vi "solar Destroy (Targets).vi"(8 "error in (no error)":errorcluster, 11 "TargetVIs":refnum<vi>[](array[refnum])) -> (0 "error out":errorcluster)   [LabVIEW 2018]
doc: "This collects all child target VIs before closing the application. This ensures all references generated by the targets are properly destroyed."
panel:
  out "VI":string
  out "VIs":string[](array[string])
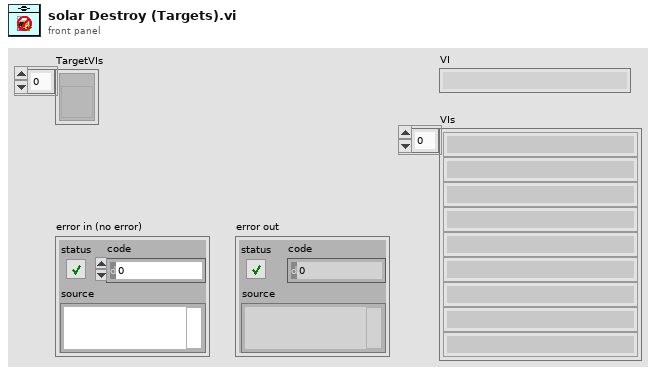
[diagram p1: front panel]
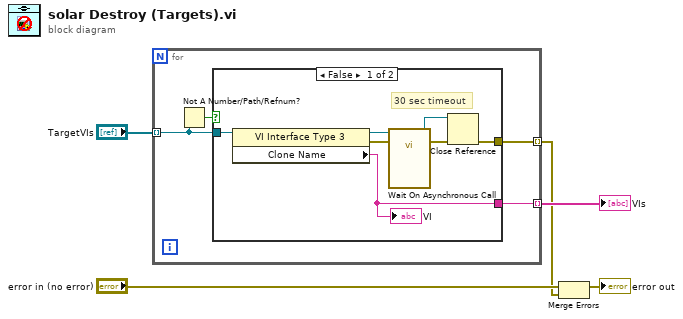
[diagram p0: block diagram]
diagram:
  n1 = for {
    tunnel: "TargetVIs" -> [w7] mode=indexing
    tunnel: [w8] -> w1 mode=indexing
    tunnel: [w9] -> w4 mode=indexing
    n2 = Not A Number/Path/Refnum?(number/path/refnum=w7) -> (NaN/Path/Refnum?=w6:bool)
    n3 = case shown="False" w6 {
      tunnel: w7 -> [w16 _]
      tunnel: [w12 _] -> w9
      tunnel: [w11 _] -> w8
      frame False {
        # "30 sec timeout"
        n4 = property class="VI Interface Type 3"(reference=w16) -> (reference out=w14:refnum<vi>, error out=w13:errorcluster, "Clone Name"=w12:string)  [unwired: 1 in]
        "VI" <- w12
        n5 = call-by-ref "Wait On Asynchronous Call"(reference=w14, error in=w13) -> (reference out=w10:refnum<vi>, error out=w15:errorcluster)  [unwired: 12 in]
        n6 = Close Reference(reference=w10, error in (no error)=w15) -> (error out=w11:errorcluster)
      }
      frame True {
      }
    }
  }
  "VIs" <- w4
  n7 = Merge Errors("error in (no error)", w1) -> (→"error out":errorcluster)
